vi "dye_experiment.vi"() -> ()   [LabVIEW 2016]
uses:
  controls/Microscope Settings.ctl
  controls/ColourCalibration.ctl
  <vilib>/DAQmx/write.llb/DAQmx Write (Digital 1D Wfm NChan NSamp).vi
  <vilib>/DAQmx/write.llb/DAQmx Write (Analog 1D Wfm NChan NSamp).vi
  <vilib>/Waveform/WDTOps.llb/WDT Number of Waveform Samples DBL.vi
  <vilib>/DAQmx/configure/timing.llb/DAQmx Timing (Sample Clock).vi
  <vilib>/Waveform/DWDTOps.llb/DWDT Uncompress Digital.vi
  <vilib>/DAQmx/miscellaneous.llb/DAQmx Fill In Error Info.vi
panel:
  out "X":dbl
  out "Z":dbl
  out "Piezo Position /um":dbl
  out "Mixed Signal Graph 2":cluster{waveform(dbl)[], digitalwaveform[]}(graph)
  out "Z":dbl
  out "X":dbl
  in  "Microscope Settings":T1={"Mode"=enum."X", "Slit"={"Scanning Mode"=1.0, "Slit Width /%"=5.0}, "Colour"=[{"Colour"={"Laser"=enum."488", "Filter"=4}, "Calibration Coordinates"={"Top Left"=[-1.5606936416184976, 4.566473988439307, 10.0], "Top Right"=[1.0404624277456644, 4.595375722543353, 10.0], "Bottom Left"=[-6.56069, 6.069364161849711, 0.0], "Bottom Right"=[6.98266, 6.069364161849711, 0.0]}}], "Focus Offset /um"=0.0, "Exposure/ms"=40.0, "Piezo Position /um"=0.0, "ROI"={"X"={"Start /px"=0.0, "Step /px"=1.0, "Range /px"=2048.0}, "Y"={"Start /px"=0.0, "Step /px"=1.0, "Range /px"=2048.0}, "Z "={"Start /um"=0.0, "Step/um"=1.0, "Range /um"=100.0}, "T "={"Start /s"=0.0, "Step /s"=1.0, "Range /s"=100.0}}, "Samples per millisecond"=100.0, "Relax/ms"=10.0, "Readout Direction"=2.0, "Trigger Source"=2.0, "Camera Delay /ms"=9.0, "Under Scan /ms"=2.0, "Slit Delay"=0.93, "Waveforms"={"Analogue Out"=[{"t0"=timestamp(0 s since 1904-01-01), "dt"=1.0, "Y"=[]}, {"t0"=timestamp(0 s since 1904-01-01), "dt"=1.0, "Y"=[]}, {"t0"=timestamp(0 s since 1904-01-01), "dt"=1.0, "Y"=[]}], "Digital Out"=[{"t0"=timestamp(0 s since 1904-01-01), "dt"=0.0, "Y"={"transitions"=[], "data"=[]}}, {"t0"=timestamp(0 s since 1904-01-01), "dt"=0.0, "Y"={"transitions"=[], "data"=[]}}, {"t0"=timestamp(0 s since 1904-01-01), "dt"=0.0, "Y"={"transitions"=[], "data"=[]}}]}} {"Focus Offset /um" scale=-2.0..2.0 scale format="%.2f"; "Under Scan /ms" min=0.0 max=10.0 step=0.05; "ROI"."T"."Range /s" min=0.0 max=10.0 step=0.05; "ROI"."T"."Step /s" min=0.0 max=10.0 step=0.05; "ROI"."T"."Start /s" min=0.0 max=10.0 step=0.05; "ROI"."X"."Range /px" min=0.0 max=10.0 step=0.05; "ROI"."X"."Step /px" min=0.0 max=10.0 step=0.05; "ROI"."X"."Start /px" min=0.0 max=10.0 step=0.05; "ROI"."Y"."Range /px" min=0.0 max=10.0 step=0.05; "ROI"."Y"."Step /px" min=0.0 max=10.0 step=0.05; "ROI"."Y"."Start /px" min=0.0 max=10.0 step=0.05; "ROI"."Z"."Range /um" min=0.0 max=10.0 step=0.05; "ROI"."Z"."Step/um" min=0.0 max=10.0 step=0.05; "ROI"."Z"."Start /um" min=0.0 max=10.0 step=0.05; "Colour"."Colour"."Filter" items=["Empty"=1, ""=2, ""=3, "561"=4, ""=5, "488"=6]; "Camera Delay /ms" min=0.0 max=10.0 step=0.05; "Trigger Source" items=["Internal"=1.0, "External"=2.0]; "Readout Direction" items=["Internal"=1.0, "External"=2.0]; "Slit"."Slit Width /%" min=0.0 max=100.0 step=0.05; "Slit"."Scanning Mode" items=["Full Frame"=1.0, "Slit Scanning"=12.0]; "Piezo Position /um" min=0.0 max=10.0 step=0.05; "Exposure/ms" min=0.0 max=10.0 step=0.05; "Relax/ms" min=1.0 max=2.0 step=1.0}
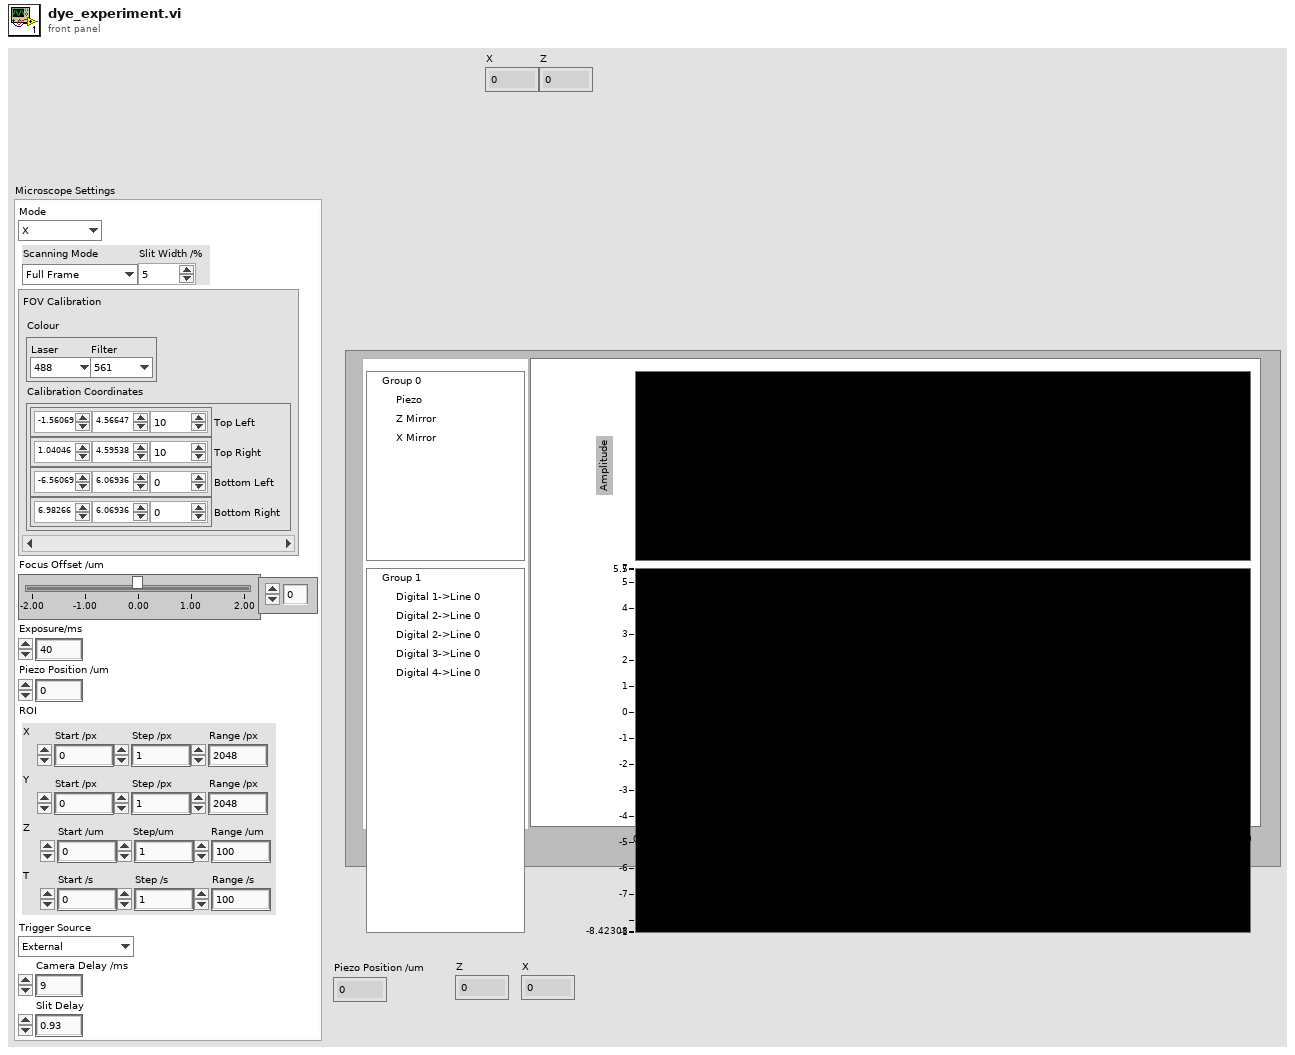
[diagram p1: front panel]
types:
  T1 = typedef "Microscope Settings.ctl" = cluster{"Mode":enum16{"Brightfield", "X", "XY", "XYZ", "XYZT", "XYZC", "Tweezers", "Virus"}, "Slit":cluster{"Scanning Mode":dbl, "Slit Width /%":dbl}, "Colour":T2, "Focus Offset /um":dbl, "Exposure/ms":dbl, "Piezo Position /um":dbl, "ROI":cluster{"X":cluster{"Start /px":dbl, "Step /px":dbl, "Range /px":dbl}, "Y":cluster{"Start /px":dbl, "Step /px":dbl, "Range /px":dbl}, "Z ":cluster{"Start /um":dbl, "Step/um":dbl, "Range /um":dbl}, "T ":cluster{"Start /s":dbl, "Step /s":dbl, "Range /s":dbl}}, "Samples per millisecond":dbl, "Relax/ms":dbl, "Readout Direction":dbl, "Trigger Source":dbl, "Camera Delay /ms":dbl, "Under Scan /ms":dbl, "Slit Delay":dbl, "Waveforms":cluster{"Analogue Out":waveform(dbl)[], "Digital Out":digitalwaveform[]}}
  T2 = typedef "ColourCalibration.ctl" = cluster{"Colour":cluster{"Laser":enum16{"Brightfield", "445", "488", "561", "647"}, "Filter":u16}, "Calibration Coordinates":cluster{"Top Left":dbl[], "Top Right":dbl[], "Bottom Left":dbl[], "Bottom Right":dbl[]}}[]
  T3 = cluster{"Analogue":refnum<k21>, "Digital":refnum<k21>}
  T4 = cluster{"Y Mirror":dbl[], "Z Mirror":dbl[], "Piezo":dbl[], "Camera":dbl[], "Laser":dbl[]}
  T5 = cluster{"Colour":cluster{"Laser":enum16{"Brightfield", "445", "488", "561", "647"}, "Filter":u16}, "Calibration Coordinates":cluster{"Top Left":dbl[], "Top Right":dbl[], "Bottom Left":dbl[], "Bottom Right":dbl[]}}
  T6 = cluster{"Top Left":dbl[], "Top Right":dbl[], "Bottom Left":dbl[], "Bottom Right":dbl[]}
  T7 = typedef "NI_Matrix.lvlib/RealMatrix.ctl" = dbl[][]
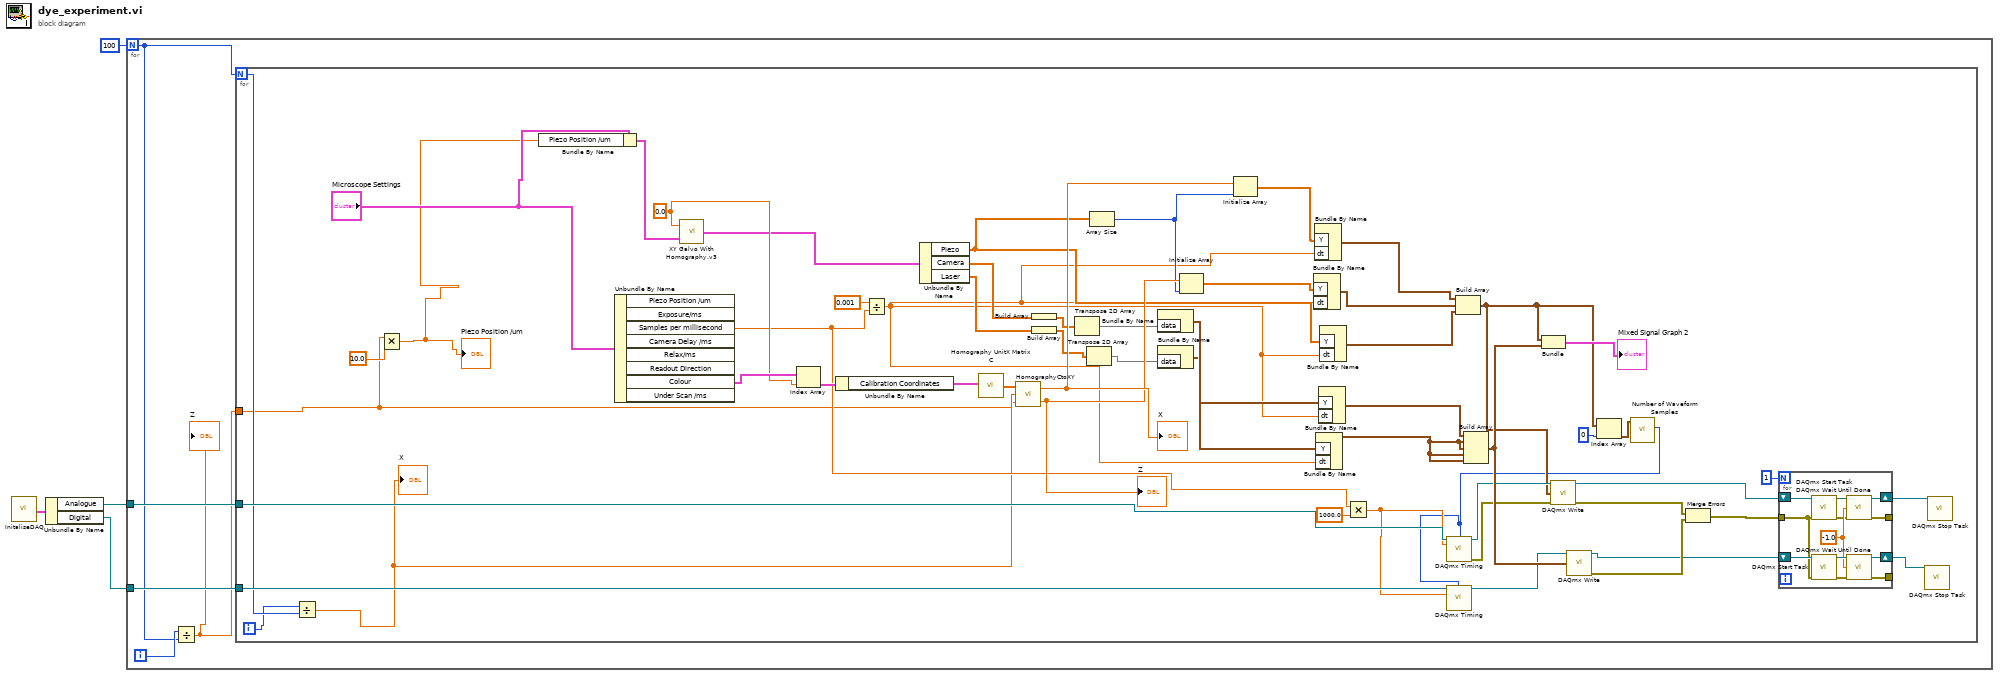
[diagram p0: block diagram]
diagram:
  n1 = call "InitaliseDAQ.vi"() -> ("Channels"=w4:T3)
  n2 = Unbundle By Name(w4) -> ("Analogue"=w3:refnum<k21>, "Digital"=w2:refnum<k21>)
  n3 = for {
    N: 100 -> [w6]
    tunnel: w3 -> [w9]
    tunnel: w2 -> [w8]
    i -> [w7]
    n4 = Divide(x=w7, y=w6) -> (x/y=w5:dbl)
    "Z" <- w5
    n5 = for {
      N: w6 -> [w16]
      tunnel: w5 -> [w10]
      tunnel: w9 -> [w38]
      tunnel: w8 -> [w36]
      i -> [w15]
      w65 = 0.0 ("Colour Channel")
      n6 = Divide(x=w15, y=w16) -> (x/y=w11:dbl)
      "X" <- w11
      n7 = Multiply(x=w10, y=10.0) -> (x*y=w14:dbl)
      "Piezo Position /um" <- w14
      n8 = Bundle By Name(cluster="Microscope Settings", "Piezo Position /um"=w14) -> (w40:T1)
      n9 = Unbundle By Name("Microscope Settings") -> ("Samples per millisecond"=w33:dbl, "Colour"=w66:T2)  [unwired: 6 out]
      n10 = call "XY Galvo With Homography.v3.vi"("Microscope Settings in"=w40, "Colour Channel"=w65) -> ("Signals"=w61:T4)
      n11 = Index Array(array=w66, index=w65) -> (element=w64:T5)
      n12 = Unbundle By Name(w64) -> ("Calibration Coordinates"=w63:T6)
      n13 = Divide(x=0.001 ("y"), y=w33) -> (x/y=w49:dbl)
      n14 = Unbundle By Name(w61) -> ("Piezo"=w50:dbl[], "Camera"=w56:dbl[], "Laser"=w55:dbl[])
      n15 = call "Homography UnitX Matrix C.vi"("input cluster"=w63) -> ("C"=w62:T7)
      n16 = call "HomographyCtoXY.vi"("Y"=w10, "X"=w11, "C"=w62) -> ("Y"=w59:dbl, "X"=w60:dbl)
      "X" <- w60
      "Z" <- w59
      n17 = Build Array(w56) -> (w45:dbl[][])
      n18 = Build Array(w55) -> (w43:dbl[][])
      n19 = Transpose 2D Array(2D array=w45) -> (transposed array=w44:dbl[][])
      n20 = Transpose 2D Array(2D array=w43) -> (transposed array=w42:dbl[][])
      n21 = Array Size(array=w50) -> (size(s)=w58:i32)
      n22 = Bundle By Name("data"=w44) -> (w54:digitaldata)  [unwired: 1 in]
      n23 = Bundle By Name("data"=w42) -> (w53:digitaldata)  [unwired: 1 in]
      n24 = Initialize Array(w59, w58) -> (w51:dbl[])
      n25 = Initialize Array(w60, w58) -> (w52:dbl[])
      n26 = Bundle By Name("Y"=w51, "dt"=w49) -> (w12:waveform(dbl))  [unwired: 1 in]
      n27 = Bundle By Name("Y"=w52, "dt"=w49) -> (w13:waveform(dbl))  [unwired: 1 in]
      n28 = Bundle By Name("Y"=w53, "dt"=w49) -> (w23:digitalwaveform)  [unwired: 1 in]
      n29 = Bundle By Name("Y"=w54, "dt"=w49) -> (w47:digitalwaveform)  [unwired: 1 in]
      n30 = Bundle By Name("Y"=w50, "dt"=w49) -> (w48:waveform(dbl))  [unwired: 1 in]
      n31 = Multiply(x=w33, y=1000.0) -> (x*y=w24:dbl)
      n32 = Build Array(w13, w12, w48) -> (w20:waveform(dbl)[])
      n33 = Build Array(w47, w23, w23, w23, w23) -> (w39:digitalwaveform[])
      n34 = Bundle(w20, w39) -> (→"Mixed Signal Graph 2":cluster{waveform(dbl)[], digitalwaveform[]})  [unwired: 1 in]
      n35 = Index Array(array=w20, index=0) -> (element=w22:waveform(dbl))
      n36 = call-poly <vilib>:"Number of Waveform Samples.vi"("waveform in"=w22) -> ("number of samples"=w19:i32)  [unwired: 8 in, 2 out]
      n37 = call-poly <vilib>:"DAQmx Timing.vi"("task/channels in"=w38, "samples per channel"=w19, "rate"=w24) -> ("task out"=w37:refnum<k21>, "error out"=w18:errorcluster)  [unwired: 11 in]
      n38 = call-poly <vilib>:"DAQmx Timing.vi"("task/channels in"=w36, "samples per channel"=w19, "rate"=w24) -> ("task out"=w35:refnum<k21>)  [unwired: 11 in, 1 out]
      n39 = call-poly <vilib>:"DAQmx Write.vi"("task/channels in"=w37, "data"=w20, "error in"=w18) -> ("task out"=w29:refnum<k21>, "error out"=w32:errorcluster)  [unwired: 10 in, 1 out]
      n40 = call-poly <vilib>:"DAQmx Write.vi"("task/channels in"=w35, "data"=w39) -> ("task out"=w28:refnum<k21>, "error out"=w31:errorcluster)  [unwired: 11 in, 1 out]
      n41 = Merge Errors(w32, w31) -> (w30:errorcluster)
      n42 = for {
        N: 1 -> [_]
        tunnel: w30 -> [w72]
        shift-right: [w75] -> w27
        shift-left: w29 -> [w78]
        shift-right: [w73] -> w26
        shift-left: w28 -> [w77]
        tunnel: [w68] -> _
        tunnel: [w67] -> _
        w71 = -1.0 ("timeout (sec)")
        n43 = call <vilib>:"DAQmx Start Task.vi"("task/channels in"=w78, "error in"=w72) -> ("task out"=w76:refnum<k21>, "error out"=w70:errorcluster)  [unwired: 12 in]
        n44 = call <vilib>:"DAQmx Start Task.vi"("task/channels in"=w77, "error in"=w72) -> ("task out"=w74:refnum<k21>, "error out"=w69:errorcluster)  [unwired: 12 in]
        n45 = call <vilib>:"DAQmx Wait Until Done.vi"("task/channels in"=w76, "timeout (sec)"=w71, "error in"=w70) -> ("task out"=w75:refnum<k21>, "error out"=w67:errorcluster)  [unwired: 11 in]
        n46 = call <vilib>:"DAQmx Wait Until Done.vi"("task/channels in"=w74, "timeout (sec)"=w71, "error in"=w69) -> ("task out"=w73:refnum<k21>, "error out"=w68:errorcluster)  [unwired: 11 in]
      }
      n47 = call <vilib>:"DAQmx Stop Task.vi"("task/channels in"=w26) -> ()  [unwired: 13 in, 2 out]
      n48 = call <vilib>:"DAQmx Stop Task.vi"("task/channels in"=w27) -> ()  [unwired: 13 in, 2 out]
    }
  }
